vi "Set VI Value Default.vi"(8 "error in (no error)":errorcluster, 9 "Default":bool, 10 "Array in":refnum<vi>, 11 "CallVIStep in":refnum<class "CallVIStep.lvclass">) -> (0 "error out":errorcluster, 3 "CallVIStep out":refnum<class "CallVIStep.lvclass">)   [LabVIEW 2015, in "CallVIStep.lvclass"]
uses:
  CallVIStep.lvclass
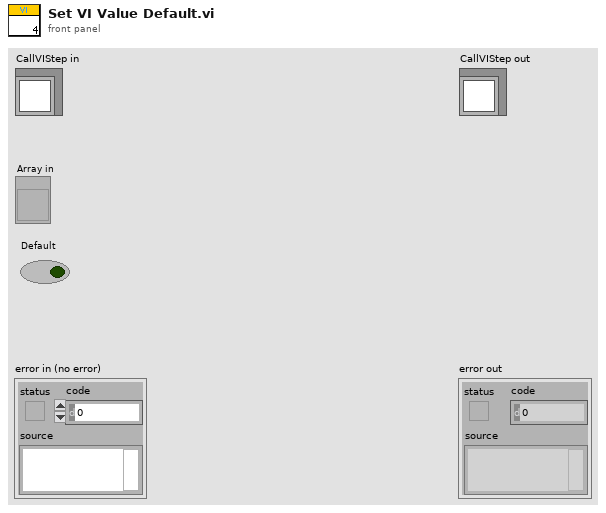
[diagram p1: front panel]
types:
  T1 = enum8{"Enabled", "Disabled", "Disabled and Grayed Out"}
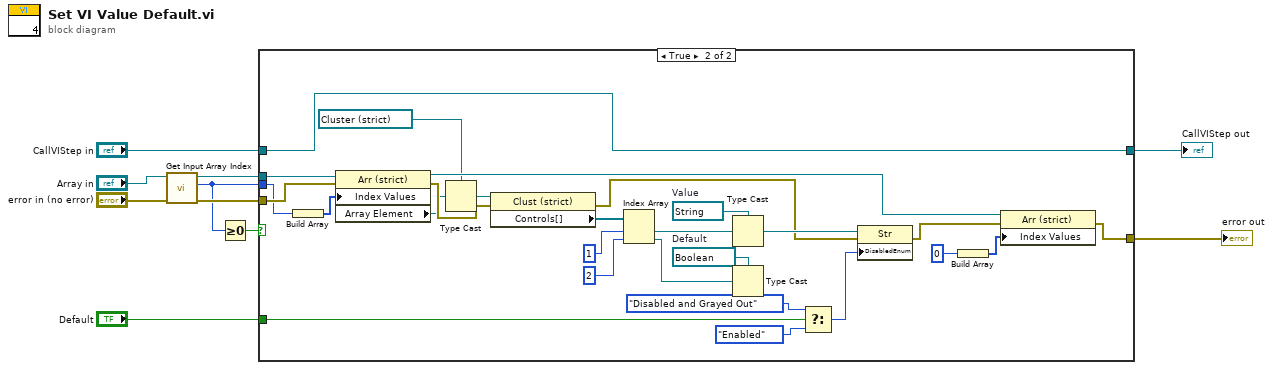
[diagram p0: block diagram]
diagram:
  n1 = call "Get Input Array Index.vi"("error in (no error)"="error in (no error)", "Array in"="Array in") -> ("error out"=w7:errorcluster, "Index"=w6:u32, "Array out"=w4:refnum<vi>)  [unwired: 7 in]
  n2 = Greater Or Equal To 0?(x=w6) -> (x >= 0?=w8:bool)
  n3 = case shown="True" w8 {
    tunnel: w7 -> [w12 w30]
    tunnel: w6 -> [_ w29]
    tunnel: "CallVIStep in" -> [w11 w21]
    tunnel: w4 -> [_ w31]
    tunnel: "Default" -> [_ w27]
    tunnel: [w12 w16] -> w2
    tunnel: [w11 w21] -> w1
    frame False {
    }
    frame True {
      w38 = refnum<vi> refnum  # Default
      w36 = refnum<vi> refnum  # Value
      n4 = Build Array(w29) -> (w14:u32[])
      n5 = property class="Arr (strict)"(reference=w31, error in=w30, "Index Values"=w14) -> (reference out=w20:refnum<vi>, error out=w23:errorcluster, "Array Element"=w15:refnum<vi>)
      n6 = Type Cast(type=refnum<vi> refnum ("Cluster"), x=w15) -> (*(type *) &x=w32:refnum<vi>)
      n7 = property class="Clust (strict)"(reference=w32, error in=w23) -> (error out=w22:errorcluster, "Controls[]"=w33:refnum<vi>[])  [unwired: 1 out]
      n8 = Index Array(array=w33, index #1=1, index #2=2) -> (element #1=w37:refnum<vi>, element #2=w39:refnum<vi>)
      n9 = Type Cast(type=w36, x=w37) -> (*(type *) &x=w28:refnum<vi>)
      n10 = Type Cast(type=w38, x=w39) -> ()  [unwired: 1 out]
      n11 = Select(t=T1."Disabled and Grayed Out" ("Disabled"), s=w27, f=T1."Enabled" ("Disabled")) -> (s? t:f=w24:T1)
      n12 = property class="Str"(reference=w28, error in=w22, "DisabledEnum"=w24) -> (error out=w17:errorcluster)  [unwired: 1 out]
      n13 = Build Array(0) -> (w18:i32[])
      n14 = property class="Arr (strict)"(reference=w20, error in=w17, "Index Values"=w18) -> (error out=w16:errorcluster)  [unwired: 1 out]
    }
  }
  "error out" <- w2
  "CallVIStep out" <- w1
